vi "Fetch New Filtered Data.vi"(7 "error in (no error)":errorcluster, 10 "Network Info in":T1 {"Last Comm Time" format="%<%H:%M:%S%3u\n%Y/%m/%d>T"; "Remote Port" format="%.0x"}) -> (0 "error out":errorcluster, 2 "Data Out":dbl[][](array[numeric]), 3 "Network Info Out":T1 {"Last Comm Time" format="%<%H:%M:%S%3u\n%Y/%m/%d>T"; "Remote Port" format="%.0x"})   [LabVIEW 2023]
doc: "Author: Scott Hannahs <sth@magnet.fsu.edu>\nCopyright 2018 Florida State University, All rights reserved."
uses:
  RT Controls/Network Info.ctl
  RT Controls/RT System Auth Level.ctl
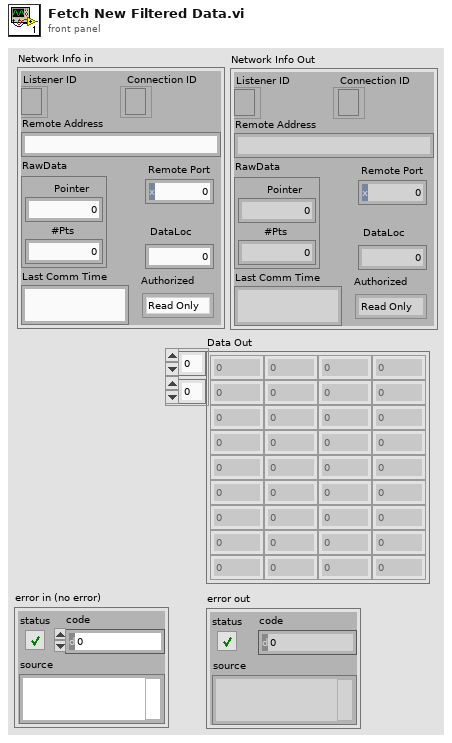
[diagram p1: front panel]
types:
  T1 = typedef "Network Info.ctl" = cluster{"Listener ID":refnum<k5>, "Connection ID":refnum<k5>, "Remote Address":string, "Remote Port":u16, "DataLoc":u32, "RawData":cluster{"#Pts":u32, "Pointer":u32}, "Last Comm Time":timestamp, "Authorized":T2}
  T2 = typedef "RT System Auth Level.ctl" = enum16{"Read Only", "Operator", "Admin"}
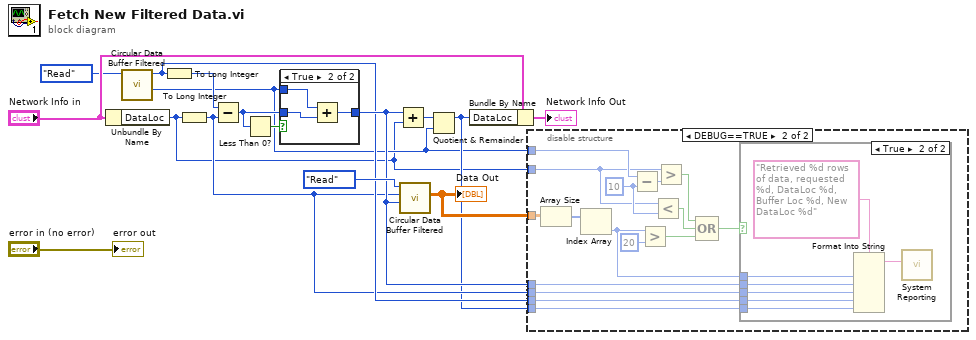
[diagram p0: block diagram]
diagram:
  n1 = Unbundle By Name("Network Info in") -> ("DataLoc"=w1:u32)
  n2 = call "Circular Data Buffer Filtered.vi"("Action"=enum16{"Initialize", "Write", "Read", "Clear"}."Read") -> ("Buffer Size"=w2:u32, "Next Write"=w6:u32)  [unwired: 8 in, 1 out]
  n3 = To Long Integer(number=w6) -> (32bit integer=w14:i32)
  n4 = To Long Integer(number=w1) -> (32bit integer=w5:i32)
  n5 = Subtract(x=w14, y=w5) -> (x-y=w16:i32)
  n6 = Less Than 0?(x=w16) -> (x < 0?=w15:bool)
  n7 = case shown="True" w15 {
    tunnel: w16 -> [w17 w20]
    tunnel: [w17 w19] -> w7
    tunnel: w2 -> [_ w18]
    frame False {
    }
    frame True {
      n8 = Add(x=w18, y=w20) -> (x+y=w19:u32)
    }
  }
  n9 = Add(x=w7, y=w1) -> (x+y=w4:u32)
  n10 = call "Circular Data Buffer Filtered.vi"("Read Size"=w7, "Read Location"=w5, "Action"=enum16{"Initialize", "Write", "Read", "Clear"}."Read") -> ("Data Out"=w8:dbl[][])  [unwired: 6 in, 2 out]
  "Data Out" <- w8
  n11 = Quotient & Remainder(x=w4, y=w2) -> (x-y*floor(x/y)=w3:u32)  [unwired: 1 out]
  n12 = Bundle By Name(cluster="Network Info in", "DataLoc"=w3) -> (→"Network Info Out":T1)
  n13 = disable-structure shown="DEBUG==TRUE" {
    disable-tunnel: w8 -> [_ w32]
    disable-tunnel: w7 -> [_ w31]
    disable-tunnel: w6 -> [_ w30]
    disable-tunnel: w5 -> [_ w29]
    disable-tunnel: w3 -> [_ w28]
    disable-tunnel: w2 -> [_ w25]
    disable-tunnel: w1 -> [_ w22]
    frame condition #0 (active) {
    }
    frame condition #1 {
      w23 = u32 10 ("y")
      n14 = Array Size(array=w32) -> (size(s)=w36:i32[])
      n15 = Index Array(array=w36) -> (element=w33:i32)  [unwired: 1 in]
      n16 = Subtract(x=w25, y=w23) -> (x-y=w26:u32)
      n17 = Greater?(x=w33, y=20) -> (0:w34:bool)
      n18 = Less?(x=w22, y=w23) -> (x < y?=w21:bool)
      n19 = Greater?(x=w22, y=w26) -> (0:w24:bool)
      n20 = Compound Arithmetic op=OR(w24, w21, w34) -> (w27:bool)
      n21 = case shown="True" w27 {
        tunnel: w33 -> [_ w43]
        tunnel: w31 -> [_ w40]
        tunnel: w29 -> [_ w39]
        tunnel: w30 -> [_ w38]
        tunnel: w28 -> [_ w37]
        frame False {
        }
        frame True {
          n22 = Format Into String(format string="Retrieved %d rows of data, requested %d, DataLoc %d, Buffer Loc %d, New DataLoc %d", w43, w40, w39, w38, w37) -> (resulting string=w41:string)  [unwired: 2 in, 1 out]
          n23 = call "System Reporting.vi"("String"=w41) -> ()  [unwired: 9 in, 2 out]
        }
      }
    }
  }
  "error out" <- "error in (no error)"
